vi "Read Scheduled.vi"(1 "scheduled time":timestamp, 2 "channel":T1) -> (5 "actual time":timestamp, 7 "element":T2={"Measurement type"=enum."Debug", "Sensor type"=enum."IFX_8in_256ch", "Identifier"="test.txt", "Open after execution?"=FALSE, "Plot after execution?"=FALSE, "Display channel"=0, "Voltage Delay (s)"=0.5, "Switch Delay (s)"=0.01, "VISA resource name source"="", "VISA resource name DMM"="", "VISA resource name LCR"="", "Compliance  Level (A)"=1e-05, "Voltage Limit (V)"=1000.0, "Data storage location"="", "Scan voltages"="", "Use source as DMM?"=FALSE, "LCR signal frequenzy (Hz)"=10000.0, "DMM device"=enum."Keithley2450", "Sampling number"=1, "Use env. sensors on"=enum."Sensirion sht1x/7x", "Switchboard Handle"=0, "Use Switchboard"=FALSE, "LCR signal voltage (V)"=10000.0, "Repeat"=1, "Scan voltages IV"="", "Scan voltages CV"="", "Hex pad numbers?"=FALSE, "Set measurement type"=enum."Debug", "Custom pad scan"="", "IV voltage Delay (s)"=0.5, "CV voltage Delay (s)"=0.5, "Needle measurement?"=FALSE, "Comments"="test.txt", "LCR signal frequenzy (kHz)"=10.0, "Compliance  Level (uA)"=10.0, "Open Correction Array"=array2304x3[6912 elements], "Current set voltage"=0.0, "Last set voltage"=0.0, "Current channel"=0, "Last OpenCorrection index"=-1, "Total curr/vltg every x steps"=10, "Current channel iteration"=0, "No CV corrections"=FALSE, "Mapfile"="", "Corrfile"="", "IV voltage file"=path "", "CV voltage file"=path "", "IV Switch Delay (s)"=0.01, "CV Switch Delay (s)"=0.01, "Invert polarity"=FALSE, "Set debug dirs"=FALSE, "Is n on p"=FALSE, "Source interlock?"=TRUE, "Voltage file used?"=FALSE, "Pad mask"="", "Mask pad above (uA)"=1.0, "LCR device"=enum."LCR_E4980", "Source device"=enum."Source_2410", "HexPlot binary path"=""} {"CV Switch Delay (s)" format="%#_13g"; "IV Switch Delay (s)" format="%#_13g"; "Last set voltage" format="%#_13g"; "Current set voltage" format="%#_13g"; "CV voltage Delay (s)" format="%#_13g"; "IV voltage Delay (s)" format="%#_13g"; "Voltage Limit (V)" format="%#_13g"; "Voltage Delay (s)" format="%#_13g"; "Switch Delay (s)" format="%#_13g"}, 8 "missed":i32)   [LabVIEW 2020, in "Tag-t'input_params.ctl'.lvlib"]
doc: "Reads a value from a Tag channel at a scheduled time."
uses:
  <extravilib>/ChannelInstances/Tag-t'input_params.ctl'.lvlib
  Desktop/HexDAQ/src/input_params.ctl
  <extravilib>/ChannelInstances/Tag-t'input_params.ctl'/))Channel.ctl
  <extravilib>/ChannelInstances/Tag-t'input_params.ctl'/Read With Abort.vi
  <extravilib>/ChannelInstances/Tag-t'input_params.ctl'/EndpointRead.vi
  <resource>/ChannelSupport/_ChannelSupport/_ChannelSupport.lvlib
  <resource>/ChannelSupport/_ChannelSupport/GetErrors/FpgaChannelWireNotSupported.xnode
panel:
  # "number of values missed\n(-1 means element is stale)"
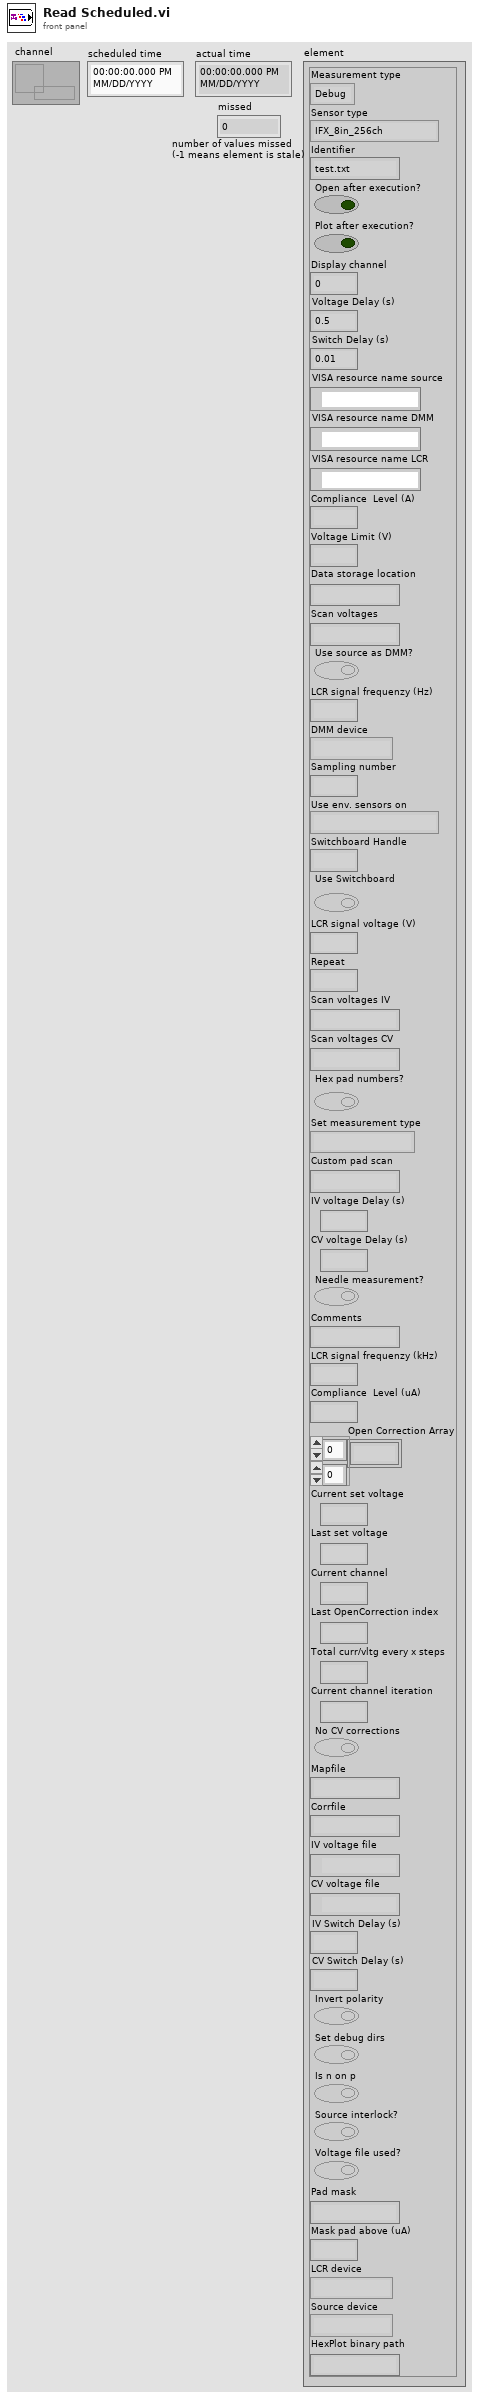
[diagram p1: front panel]
types:
  T1 = typedef "Tag-t'input_params.ctl'.lvlib/))Channel.ctl" = refnum<queue>
  T2 = typedef "input_params.ctl" = cluster{"Measurement type":enum16{"IV", "CV", "Debug", "Test_contact"}, "Sensor type":enum16{"HPK_6in_135ch", "HPK_8in_271ch", "IFX_8in_256ch", "Diode", "HPK_6in_239ch", "Full_Matrix", "HPK_8in_271ch_full", "HPK_8in_198ch", "LumiCal", "HPK_8in_444ch", "HPK_8in_198ch_2019"}, "Identifier":string, "Open after execution?":bool, "Plot after execution?":bool, "Display channel":i32, "Voltage Delay (s)":dbl, "Switch Delay (s)":dbl, "VISA resource name source":refnum<visa-resource-name>, "VISA resource name DMM":refnum<visa-resource-name>, "VISA resource name LCR":refnum<visa-resource-name>, "Compliance  Level (A)":dbl, "Voltage Limit (V)":dbl, "Data storage location":string, "Scan voltages":string, "Use source as DMM?":bool, "LCR signal frequenzy (Hz)":dbl, "DMM device":enum16{"Keithley2001", "Keithley2450", "Keithley2410", "Keithley6485", "Keithley6487", "Keithley6517"}, "Sampling number":i32, "Use env. sensors on":enum16{"Sensirion sht1x/7x", "Switch Matrix", "Probecard"}, "Switchboard Handle":u32, "Use Switchboard":bool, "LCR signal voltage (V)":dbl, "Repeat":i32, "Scan voltages IV":string, "Scan voltages CV":string, "Hex pad numbers?":bool, "Set measurement type":enum16{"IV", "CV", "Debug", "Test_contact", "IV+CV"}, "Custom pad scan":string, "IV voltage Delay (s)":dbl, "CV voltage Delay (s)":dbl, "Needle measurement?":bool, "Comments":string, "LCR signal frequenzy (kHz)":dbl, "Compliance  Level (uA)":dbl, "Open Correction Array":dbl[][], "Current set voltage":dbl, "Last set voltage":dbl, "Current channel":i32, "Last OpenCorrection index":i32, "Total curr/vltg every x steps":i32, "Current channel iteration":i32, "No CV corrections":bool, "Mapfile":string, "Corrfile":string, "IV voltage file":path, "CV voltage file":path, "IV Switch Delay (s)":dbl, "CV Switch Delay (s)":dbl, "Invert polarity":bool, "Set debug dirs":bool, "Is n on p":bool, "Source interlock?":bool, "Voltage file used?":bool, "Pad mask":string, "Mask pad above (uA)":dbl, "LCR device":enum16{"LCR_E4980", "AGILENT_4263X"}, "Source device":enum16{"Source_2410", "Source_6487"}, "HexPlot binary path":string}
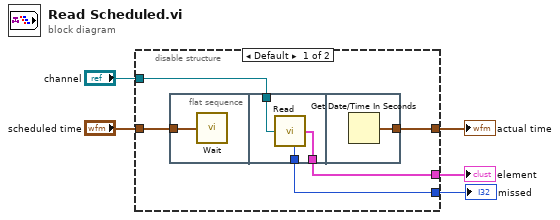
[diagram p0: block diagram]
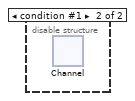
[diagram p2: hidden frame]
diagram:
  n1 = disable-structure shown="Default" {
    disable-tunnel: "scheduled time" -> [w10 _]
    disable-tunnel: [w9 _] -> w4
    disable-tunnel: "channel" -> [w8 _]
    disable-tunnel: [w7 _] -> w2
    disable-tunnel: [w6 _] -> w1
    frame condition #0 (active) {
      n2 = flat-sequence {
        tunnel: w10 -> [w11]
        tunnel: w8 -> [w14]
        tunnel: [w13] -> w7
        tunnel: [w12] -> w6
        tunnel: [w15] -> w9
        frame #0 {
          n3 = call <resource>:"Wait.vi"("desired time"=w11) -> ()  [unwired: 2 out]
        }
        frame #1 {
          n4 = call <extravilib>:"Read.vi"("channel"=w14) -> ("missed"=w12:i32, "element"=w13:T2)  [unwired: 1 in]
        }
        frame #2 {
          n5 = Get Date/Time In Seconds() -> (seconds since 1Jan1904=w15:timestamp)
        }
      }
    }
    frame condition #1 {
      n6 = xnode "Channel"() -> ()
    }
  }
  "element" <- w2
  "actual time" <- w4
  "missed" <- w1
